vi "_TangoPing.vi"(2 "error in":errorcluster, 3 "device name":string) -> (0 "error out":errorcluster, 1 "rrt":i32)   [LabVIEW 2014, in "tango.lvlib"]
uses:
  tango.lvlib
  tango_binding.so
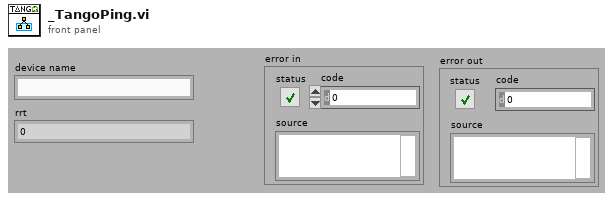
[diagram p1: front panel]
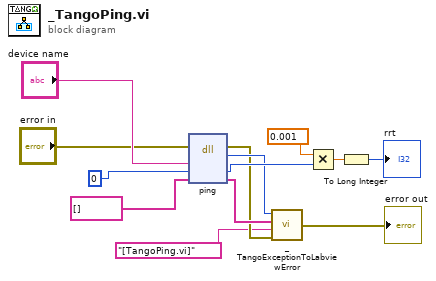
[diagram p0: block diagram]
diagram:
  n1 = dll-call lib="tango_binding.*" fn="ping"(error in="error in", "dev_name"="device name", "rtt"=0, "error_stack"=string[] [] ("Error Stack")) -> (error out=w2:errorcluster, "return type"=w5:i32, "rtt"=w13:u32, "error_stack"=w4:string[])  [unwired: 3 in, 1 out]
  n2 = call "_TangoExceptionToLabviewError.vi"("error in"=w2, "location"="[TangoPing.vi]", "error stack"=w4, "error code"=w5) -> ("error out"=→"error out":errorcluster)
  n3 = Multiply(x=0.001, y=w13) -> (x*y=w10:dbl)
  n4 = To Long Integer(number=w10) -> (32bit integer=→"rrt":i32)
